vi "401_Selected_User.vi"(8 "error in (no error)":errorcluster, 10 "User Name":string, 11 "connection in":T1) -> (0 "error Out":errorcluster, 3 "Data_Table":string[][](array[string]))   [LabVIEW 2015]
uses:
  <vilib>/addons/database/Connection.llb/Conn ObjectReference.ctl
  <vilib>/addons/database/NI_Database_API.lvlib
panel:
  out "connection out":T1
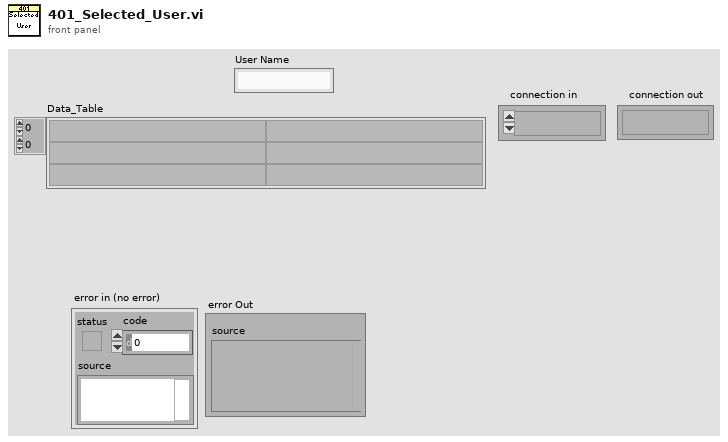
[diagram p1: front panel]
types:
  T1 = typedef "NI_Database_API.lvlib/Conn ObjectReference.ctl" = refnum<k1>
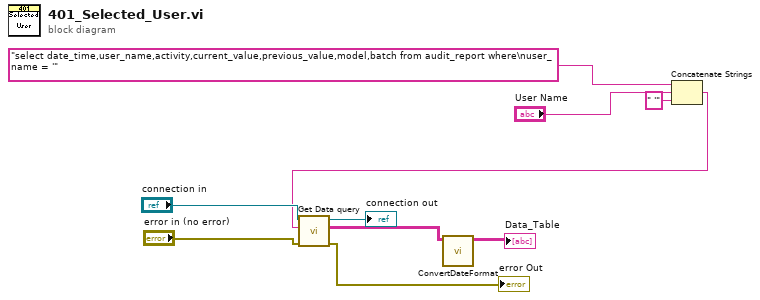
[diagram p0: block diagram]
diagram:
  n1 = Concatenate Strings("select date_time,user_name,activity,current_value,previous_value,model,batch from audit_report where\nuser_name = '" ("string"), "User Name", " '" ("string")) -> (w3:string)
  n2 = call "Get Data query.vi"("error in"="error in (no error)", "SQL query"=w3, "connection reference"="connection in") -> ("error Out"=→"error Out":errorcluster, "Data_Table"=w2:string[][], "connection reference"=→"connection out":T1)  [unwired: 6 in]
  n3 = call "ConvertDateFormat.vi"("DataIn"=w2) -> ("DataOut"=→"Data_Table":string[][])  [unwired: 10 in]
